vi "GlobalVars.vi"() -> ()   [LabVIEW 2017]
panel:
  out "ScaleAngleOffset":dbl
  out "ScaleAngle":dbl=-999.0
  out "MatchData":cluster{"MatchTime":sgl, "CANUtilization":sgl}
  out "ClimberFault":bool
  out "ArmFault":bool
  out "ArmLength":dbl
  out "HasCube":bool
  out "ArmAngle":dbl
  out "CameraIP":string="10.1.95.11"
  in  "ElevatorPositionReq":dbl(slide) scale=0.0..100.0
  out "ElevatorPositionAct":dbl(slide) scale=0.0..100.0
  out "RightDrive3Current":dbl
  out "RightDrive2Current":dbl
  out "RightDriveOutput":dbl
  out "RightDrive1Current":dbl
  out "RightDriveVel":dbl
  out "RightDrivePos":dbl
  out "LeftDrive3Current":dbl
  out "LeftDrive2Current":dbl
  out "LeftDriveOutput":dbl
  out "LeftDrive1Current":dbl
  out "LeftDriveVel":dbl
  out "LeftDrivePos":dbl
  out "ElevatorFault":bool
  out "IntakeOnChris":bool
  out "IntakeOnJake":bool
  out "TurretPos":dbl(slide)=2.0140350877192983 scale=-2.0..6.0 scale format="%#_2e"
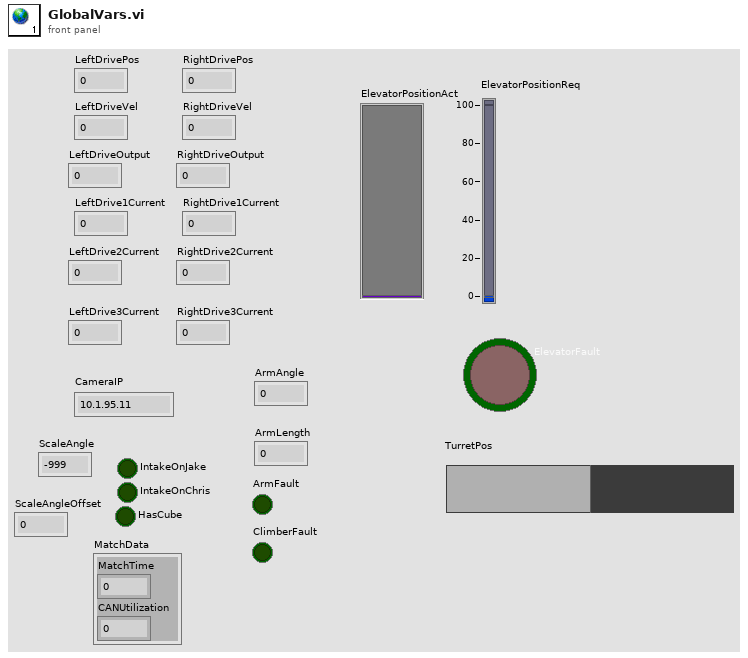
[diagram p1: front panel]
diagram:
